vi "GetAutomaticParameterMode.vi"(7 "Auto Parameter":T2, 8 "error in (no error)":errorcluster, 11 "CameraStream in":refnum<class "CameraStream.lvclass">) -> (0 "error out":errorcluster, 1 "Is Supported":bool, 2 "Automatic Parameter Mode":T1, 3 "CameraStream (Duplicate)":refnum<class "CameraStream.lvclass">)   [LabVIEW 2020, in "g_ar_toolkit.capture.lvlib" / "CameraStream.lvclass"]
uses:
  CameraStream.lvclass
  Camera Automatic Parameters.ctl
  Camera Automatic Parameter Mode.ctl
  CameraStream.lvclass/CameraStream.ctl
  g_ar_toolkit.common/g_ar_toolkit.common.lvlib
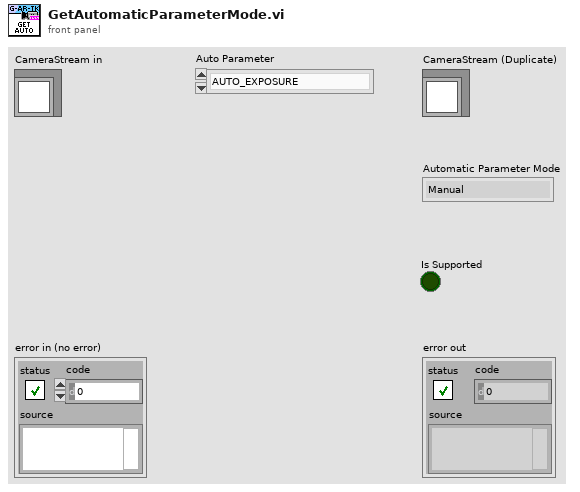
[diagram p1: front panel]
types:
  T1 = typedef "g_ar_toolkit.capture.lvlib/CameraStream.lvclass/Camera Automatic Parameter Mode.ctl" = enum16{"Manual", "Automatic"}
  T2 = typedef "g_ar_toolkit.capture.lvlib/CameraStream.lvclass/Camera Automatic Parameters.ctl" = enum16{"AUTO_EXPOSURE", "AUTO_FOCUS", "AUTO_WHITE_BALANCE", "AUTO_GAIN"}
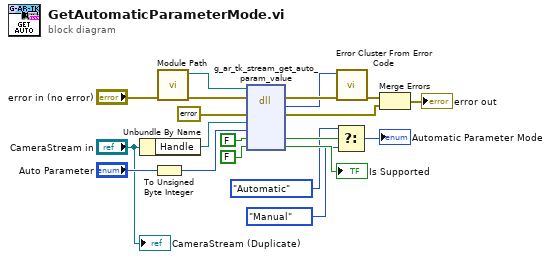
[diagram p0: block diagram]
diagram:
  n1 = Unbundle By Name("CameraStream in") -> ("Handle"=w16:refnum<data-value>)
  n2 = To Unsigned Byte Integer(number="Auto Parameter") -> (unsigned 8bit integer=w10:u8)
  n3 = call "Module Path.vi"("error in (no error)"="error in (no error)") -> ("error out"=w2:errorcluster, "Path"=w1:path)  [unwired: 9 in]
  n4 = dll-call lib="?" fn="g_ar_tk_stream_get_auto_param_value" ("g_ar_toolkit.*.*:g_ar_tk_stream_capture_next")(path in=w1, error in=w2, "error_cluster"=errorcluster {"status"=FALSE, "code"=0, "source"=""} ("error constant"), "EDVR_strm"=w16, "parameter"=w10, "is_automatic"=FALSE, "is_supported"=FALSE) -> (error out=w15:errorcluster, "MgErr"=w14:i32, "error_cluster"=w12:errorcluster, "is_automatic"=w7:bool, "is_supported"=→"Is Supported":bool)  [unwired: 3 in, 1 out]
  n5 = Select(t=Camera_Automatic_Parameter_Mode."Automatic" ("Automatic Parameter Mode"), s=w7, f=Camera_Automatic_Parameter_Mode."Manual") -> (s? t:f=→"Automatic Parameter Mode":T1)
  n6 = call <vilib>:"Error Cluster From Error Code.vi"("error in (no error)"=w15, "error code (0)"=w14) -> ("error out"=w13:errorcluster)  [unwired: 7 in]
  n7 = Merge Errors(w13, w12) -> (→"error out":errorcluster)
  "CameraStream (Duplicate)" <- "CameraStream in"
